vi "GenerateGraph.vi"() -> ()   [LabVIEW 2019]
uses:
  Global 2.vi
  <vilib>/Utility/file.llb/Read Delimited Spreadsheet (DBL).vi
panel:
  out "Vibration Z":cluster{"all rows":dbl[], "all rows":dbl[]}[](graph)
  out "Vibration Y":cluster{"all rows":dbl[], "all rows":dbl[]}[](graph)
  out "Vibration X":cluster{"all rows":dbl[], "all rows":dbl[]}[](graph)
  in  "?":bool
  in  "?":bool
  out "Current":cluster{"all rows":dbl[], "all rows":dbl[]}[](graph)
  in  "Interval":i32=4
  # "Graph Moving Average"
  # "Interval"
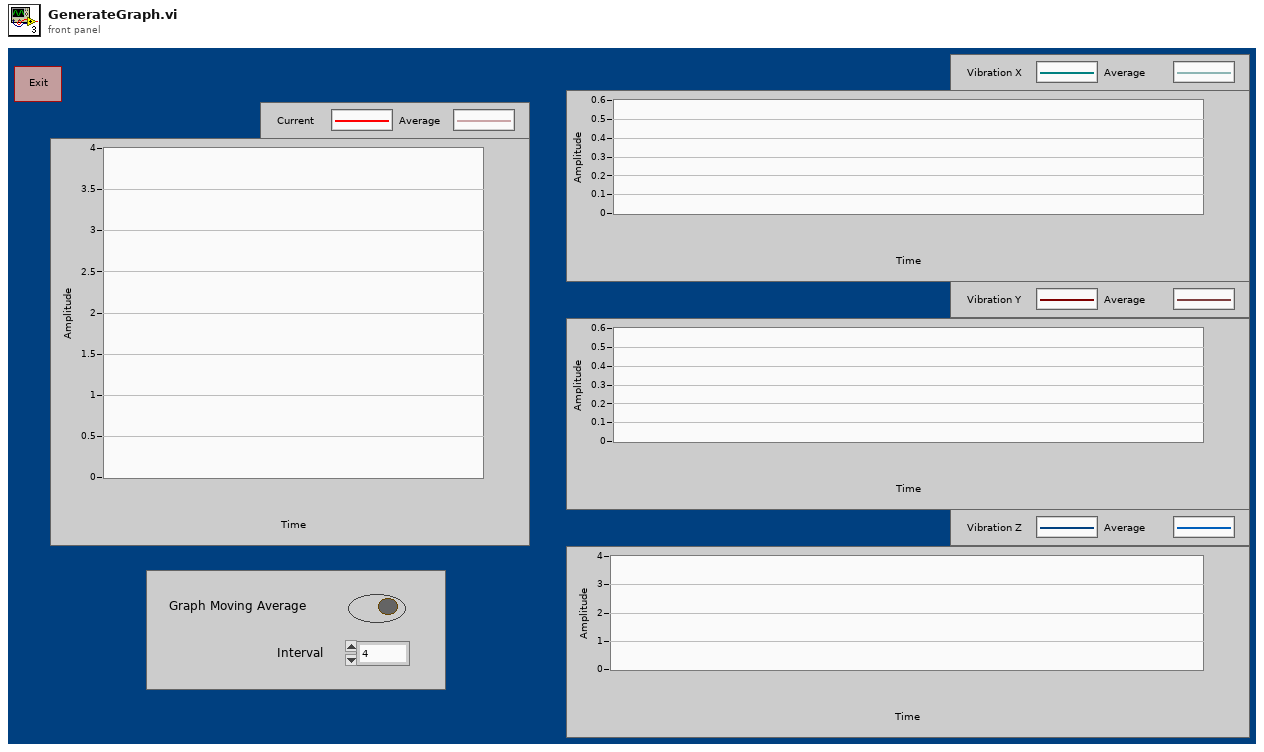
[diagram p1: front panel]
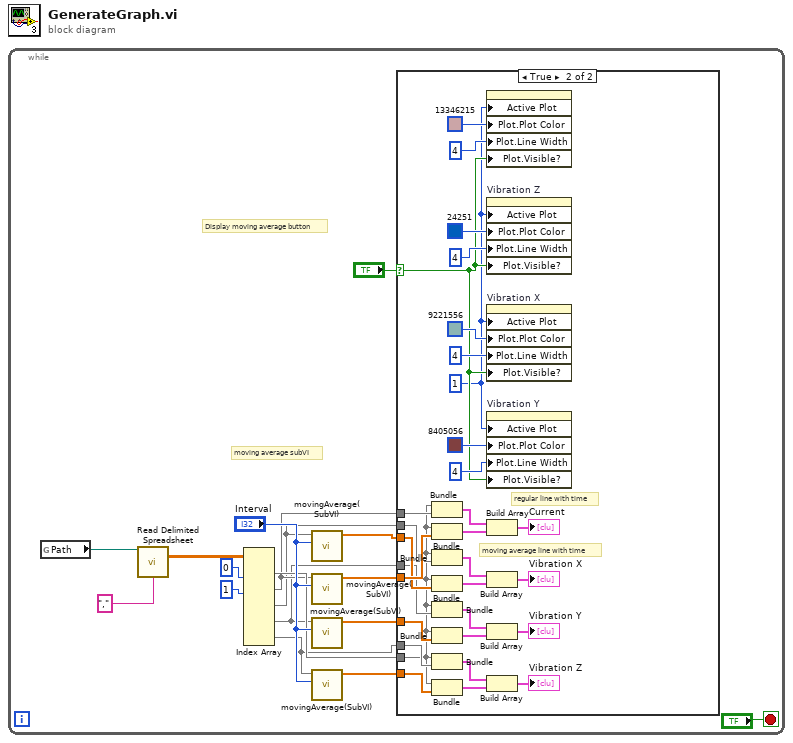
[diagram p0: block diagram]
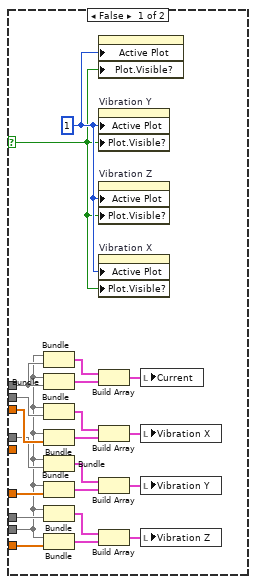
[diagram p2: hidden frame]
diagram:
  n1 = while {
    stop <- "?" stop-if-true
    # "moving average subVI"
    # "Display moving average button"
    n2 = global read "Global 2.vi" "Path"() -> (w10:path)
    n3 = call-poly <vilib>:"Read Delimited Spreadsheet.vi"("file path (dialog if empty)"=w10, "delimiter (\\t)"="," ("delimiter (\\t)")) -> ("all rows"=w9:dbl[][])  [unwired: 8 in, 5 out]
    n4 = Index Array(array=w9, index (col) #1=0 ("disabled index (col)"), index (col) #2=1 ("index (col)")) -> (element #1=w5:dbl[], element #2=w4:dbl[], element #3=w3:dbl[], element #4=w2:dbl[], element #5=w1:dbl[])  [unwired: 8 in]
    n5 = call "movingAverage(SubVI).vi"("length"="Interval", "all rows"=w3) -> ("Array"=w14:dbl[])  [unwired: 9 in]
    n6 = call "movingAverage(SubVI).vi"("length"="Interval", "all rows"=w4) -> ("Array"=w15:dbl[])  [unwired: 9 in]
    n7 = call "movingAverage(SubVI).vi"("length"="Interval", "all rows"=w2) -> ("Array"=w13:dbl[])  [unwired: 9 in]
    n8 = call "movingAverage(SubVI).vi"("length"="Interval", "all rows"=w1) -> ("Array"=w11:dbl[])  [unwired: 9 in]
    n9 = case shown="True" "?" {
      selector: "?" -> [w24 w42]
      tunnel: w5 -> [w19 w43]
      tunnel: w4 -> [w39 w70]
      tunnel: w15 -> [_ w69]
      tunnel: w3 -> [w33 w62]
      tunnel: w14 -> [w32 w61]
      tunnel: w13 -> [w27 w54]
      tunnel: w2 -> [w26 w53]
      tunnel: w1 -> [w21 w45]
      tunnel: w11 -> [w20 w44]
      frame False {
        w25 = u32 1 ("Active Plot")
        n10 = Bundle("all rows"=w19, "all rows"=w39) -> (w37:cluster{"all rows":dbl[], "all rows":dbl[]})  [unwired: 1 in]
        n11 = Bundle("all rows"=w19, "all rows"=w39) -> (w36:cluster{"all rows":dbl[], "all rows":dbl[]})  [unwired: 1 in]
        n12 = Bundle("all rows"=w19, "all rows"=w33) -> (w35:cluster{"all rows":dbl[], "all rows":dbl[]})  [unwired: 1 in]
        n13 = Bundle("all rows"=w19, "Array"=w32) -> (w34:cluster{"all rows":dbl[], "Array":dbl[]})  [unwired: 1 in]
        n14 = Bundle("all rows"=w19, "all rows"=w26) -> (w30:cluster{"all rows":dbl[], "all rows":dbl[]})  [unwired: 1 in]
        n15 = Bundle("all rows"=w19, "Array"=w27) -> (w29:cluster{"all rows":dbl[], "Array":dbl[]})  [unwired: 1 in]
        n16 = Bundle("all rows"=w19, "all rows"=w21) -> (w23:cluster{"all rows":dbl[], "all rows":dbl[]})  [unwired: 1 in]
        n17 = Bundle("all rows"=w19, "Array"=w20) -> (w22:cluster{"all rows":dbl[], "Array":dbl[]})  [unwired: 1 in]
        n18 = property on="Current" class="XYGraph (strict)"("Active Plot"=w25, "Plot.Visible?"=w24) -> ()  [unwired: 2 in, 2 out]
        n19 = property on="Vibration Y" class="XYGraph (strict)"("Active Plot"=w25, "Plot.Visible?"=w24) -> ()  [unwired: 2 in, 2 out]
        n20 = property on="Vibration Z" class="XYGraph (strict)"("Active Plot"=w25, "Plot.Visible?"=w24) -> ()  [unwired: 2 in, 2 out]
        n21 = property on="Vibration X" class="XYGraph (strict)"("Active Plot"=w25, "Plot.Visible?"=w24) -> ()  [unwired: 2 in, 2 out]
        n22 = Build Array(w37, w36) -> (w38:cluster{"all rows":dbl[], "all rows":dbl[]}[])
        n23 = Build Array(w35, w34) -> (w31:cluster{"all rows":dbl[], "Array":dbl[]}[])
        n24 = Build Array(w30, w29) -> (w28:cluster{"all rows":dbl[], "Array":dbl[]}[])
        n25 = Build Array(w23, w22) -> (w18:cluster{"all rows":dbl[], "Array":dbl[]}[])
        n26 = local write "Current"(w38) -> ()
        n27 = local write "Vibration X"(w31) -> ()
        n28 = local write "Vibration Y"(w28) -> ()
        n29 = local write "Vibration Z"(w18) -> ()
      }
      frame True {
        w41 = u32 1 ("Active Plot")
        # "moving average line with time"
        # "regular line with time"
        n30 = Bundle("all rows"=w43, "all rows"=w70) -> (w65:cluster{"all rows":dbl[], "all rows":dbl[]})  [unwired: 1 in]
        n31 = Bundle("all rows"=w43, "Array"=w69) -> (w66:cluster{"all rows":dbl[], "Array":dbl[]})  [unwired: 1 in]
        n32 = Bundle("all rows"=w43, "all rows"=w62) -> (w63:cluster{"all rows":dbl[], "all rows":dbl[]})  [unwired: 1 in]
        n33 = Bundle("all rows"=w43, "Array"=w61) -> (w60:cluster{"all rows":dbl[], "Array":dbl[]})  [unwired: 1 in]
        n34 = Bundle("all rows"=w43, "all rows"=w53) -> (w52:cluster{"all rows":dbl[], "all rows":dbl[]})  [unwired: 1 in]
        n35 = Bundle("all rows"=w43, "Array"=w54) -> (w57:cluster{"all rows":dbl[], "Array":dbl[]})  [unwired: 1 in]
        n36 = Bundle("all rows"=w43, "all rows"=w45) -> (w47:cluster{"all rows":dbl[], "all rows":dbl[]})  [unwired: 1 in]
        n37 = Bundle("all rows"=w43, "Array"=w44) -> (w50:cluster{"all rows":dbl[], "Array":dbl[]})  [unwired: 1 in]
        n38 = property on="Current" class="XYGraph (strict)"("Active Plot"=w41, "Plot.Plot Color"=u32 13346215, "Plot.Line Width"=u8 4, "Plot.Visible?"=w42) -> ()  [unwired: 2 in, 2 out]
        n39 = property on="Vibration Z" class="XYGraph (strict)"("Active Plot"=w41, "Plot.Plot Color"=u32 24251, "Plot.Line Width"=u8 4, "Plot.Visible?"=w42) -> ()  [unwired: 2 in, 2 out]
        n40 = property on="Vibration X" class="XYGraph (strict)"("Active Plot"=w41, "Plot.Plot Color"=u32 9221556, "Plot.Line Width"=u8 4, "Plot.Visible?"=w42) -> ()  [unwired: 2 in, 2 out]
        n41 = property on="Vibration Y" class="XYGraph (strict)"("Active Plot"=w41, "Plot.Plot Color"=u32 8405056, "Plot.Line Width"=u8 4, "Plot.Visible?"=w42) -> ()  [unwired: 2 in, 2 out]
        n42 = Build Array(w65, w66) -> (→"Current":cluster{"all rows":dbl[], "Array":dbl[]}[])
        n43 = Build Array(w63, w60) -> (→"Vibration X":cluster{"all rows":dbl[], "Array":dbl[]}[])
        n44 = Build Array(w52, w57) -> (→"Vibration Y":cluster{"all rows":dbl[], "Array":dbl[]}[])
        n45 = Build Array(w47, w50) -> (→"Vibration Z":cluster{"all rows":dbl[], "Array":dbl[]}[])
      }
    }
  }
